vi "runAnalyer.vi"(8 "error in (no error)":errorcluster, 10 "closeEvent":refnum<user-event>, 11 "ImageAnalyser in":refnum<class "ImageAnalyser.lvclass">) -> (0 "error out":errorcluster, 3 "ImageAnalyser out":refnum<class "ImageAnalyser.lvclass">)   [LabVIEW 2009, in "Tools.lvlib" / "Imaging.lvlib" / "ImageAnalyser.lvclass"]
uses:
  ImageAnalyser.lvclass
panel:
  in  "stop":bool
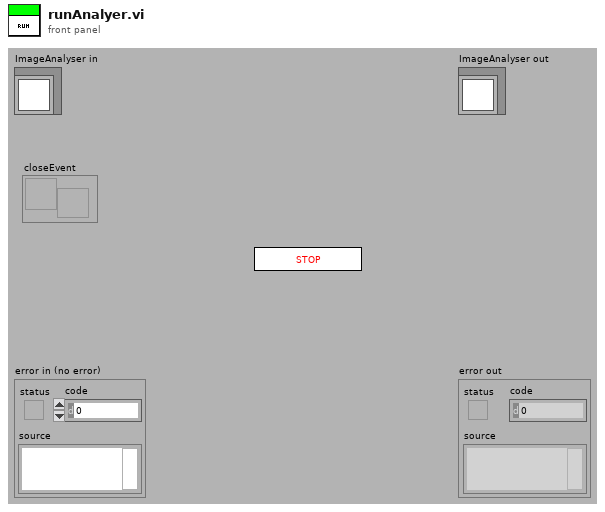
[diagram p1: front panel]
types:
  T1 = cluster{"ImageName":string, "ImageArray":sgl[][]}
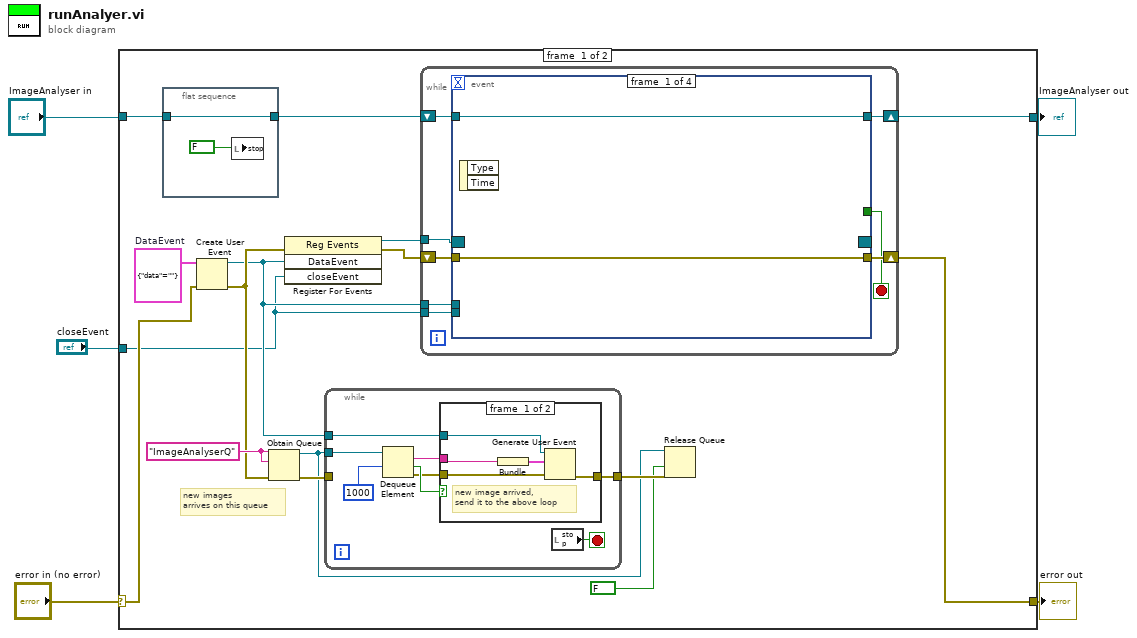
[diagram p0: block diagram]
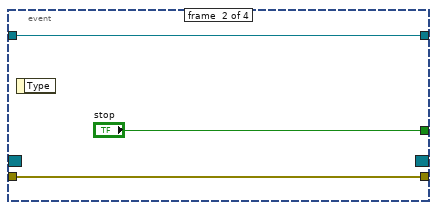
[diagram p2: hidden frame]
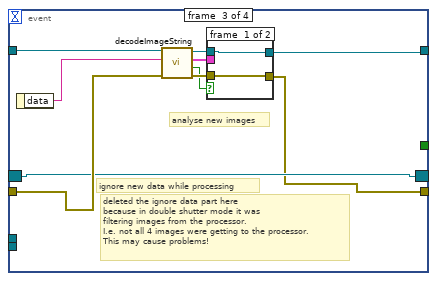
[diagram p3: hidden frame]
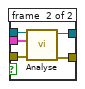
[diagram p4: hidden frame]
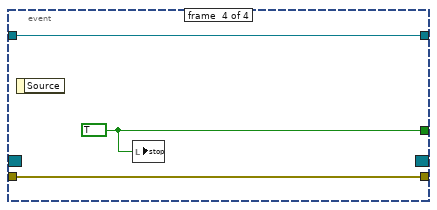
[diagram p5: hidden frame]
diagram:
  n1 = case shown="No Error" "error in (no error)" {
    selector: "error in (no error)" -> [w13 w72]
    tunnel: [w6 w72] -> w4
    tunnel: [w17 w71] -> w2
    tunnel: "ImageAnalyser in" -> [w9 w71]
    tunnel: "closeEvent" -> [w7 _]
    frame #0 {
      w15 = cluster{"data":string} {"data"=""}  # DataEvent
      w16 = "ImageAnalyserQ"
      # "new images\narrives on this queue"
      n2 = flat-sequence {
        tunnel: [w23] -> w10
        tunnel: w9 -> [w23]
        frame #0 {
          n3 = local write "stop"(FALSE) -> ()
        }
      }
      n4 = Create User Event(user event datatype=w15, error in=w13) -> (user event=w8:refnum<user-event>, error out=w12:errorcluster)
      n5 = Obtain Queue(name (unnamed)=w16, element data type=w16, error in (no error)=w12) -> (queue out=w19:refnum<queue>, error out=w21:errorcluster)  [unwired: 2 in, 1 out]
      n6 = register-events(error in=w12, w8, w7) -> (reference out=w14:refnum<event-registration>, error out=w11:errorcluster)  [unwired: 1 in]
      n7 = while {
        tunnel: w19 -> [w64]
        tunnel: w21 -> [_]
        tunnel: [w61] -> w20
        tunnel: w8 -> [w58]
        stop <- w60 stop-if-true
        n8 = Dequeue Element(queue=w64, timeout in ms (-1)=1000) -> (element=w59:string, timed out?=w63:bool, error out=w62:errorcluster)  [unwired: 1 in, 1 out]
        n9 = case shown="False" w63 {
          tunnel: w62 -> [w69 w70]
          tunnel: [w68 w70] -> w61
          tunnel: w59 -> [w67 _]
          tunnel: w58 -> [w66 _]
          frame #0 {
            # "new image arrived, \nsend it to the above loop"
            n10 = Bundle(w67) -> (w65:cluster{string})  [unwired: 1 in]
            n11 = Generate User Event(user event=w66, event data cluster=w65, error in=w69) -> (error out=w68:errorcluster)  [unwired: 1 out]
          }
          frame #1 {
            # "timeout"
          }
        }
        n12 = local read "stop"() -> (w60:bool)
      }
      n13 = while {
        shift-right: [w31] -> w17
        shift-left: w10 -> [w30]
        tunnel: w14 -> [w29]
        shift-right: [w27] -> w6
        shift-left: w11 -> [w28]
        tunnel: w8 -> [w25]
        tunnel: w7 -> [w24]
        stop <- w26 stop-if-true
        n14 = event shown="[2] <DataEvent>: User Event" {
          selector: w29 -> [_ _ w38 _]
          dyn-events: [_ _ w38 _] -> _
          timeout: _ -> [_ _ _ _]
          tunnel: [w33 w34 w43 w56] -> w31
          tunnel: w30 -> [w33 w34 w46 w56]
          tunnel: w28 -> [w32 w36 w39 w55]
          tunnel: [w32 w36 w37 w55] -> w27
          tunnel: [_ "stop" _ w54] -> w26
          tunnel: w25 -> [_ _ _ _]
          tunnel: w24 -> [_ _ _ _]
          event #0 {
            n15 = event-data() -> ()  [unwired: 1 in, 2 out]
          }
          event #1 {
            n16 = event-data() -> ()  [unwired: 1 in, 1 out]
          }
          event #2 {
            # "deleted the ignore data part here\nbecause in double shutter mode it was \nfiltering images from the processor.\nI.e. not all 4 images were getting to the processor.\nThis may cause problems!"
            # "ignore new data while processing"
            # "analyse new images"
            n17 = event-data() -> ("data"=w45:string)  [unwired: 1 in]
            n18 = call "decodeImageString.vi"("error in (no error)"=w39, "encodedImage"=w45, "ImageAnalyser in"=w46) -> ("error out"=w42:errorcluster, "isImage?"=w41:bool, "ImageData"=w40:T1, "ImageAnalyser out"=w44:refnum<class "ImageAnalyser.lvclass">)  [unwired: 5 in]
            n19 = case shown="True" w41 {
              tunnel: w44 -> [w48 w53]
              tunnel: [w48 w52] -> w43
              tunnel: w42 -> [w47 w51]
              tunnel: [w47 w50] -> w37
              tunnel: w40 -> [_ w49]
              frame #0 {
              }
              frame #1 {
                n20 = call-dynamic "Analyse.vi"("error in (no error)"=w51, "ImageData"=w49, "ImageAnalyser in"=w53) -> ("error out"=w50:errorcluster, "ImageAnalyser out"=w52:refnum<class "ImageAnalyser.lvclass">)  [unwired: 7 in]
              }
            }
          }
          event #3 {
            w54 = TRUE
            n21 = event-data() -> ()  [unwired: 1 in, 1 out]
            n22 = local write "stop"(w54) -> ()
          }
        }
      }
      n23 = Release Queue(queue=w19, force destroy? (F)=FALSE, error in (no error)=w20) -> ()  [unwired: 3 out]
    }
    frame #1 {
    }
  }
  "error out" <- w4
  "ImageAnalyser out" <- w2
